vi "Parse ERD Write Expected Data.vi"(0 "Write ERD List":T1[](array[typedef]) {"ERD Number" format="%.0x"}, 11 "Error In":errorcluster) -> (8 "Expected Data":string, 15 "Error Out":errorcluster)   [LabVIEW 2023]
uses:
  type defs/ERD Write Data In.ctl
  type defs/Data Type.ctl
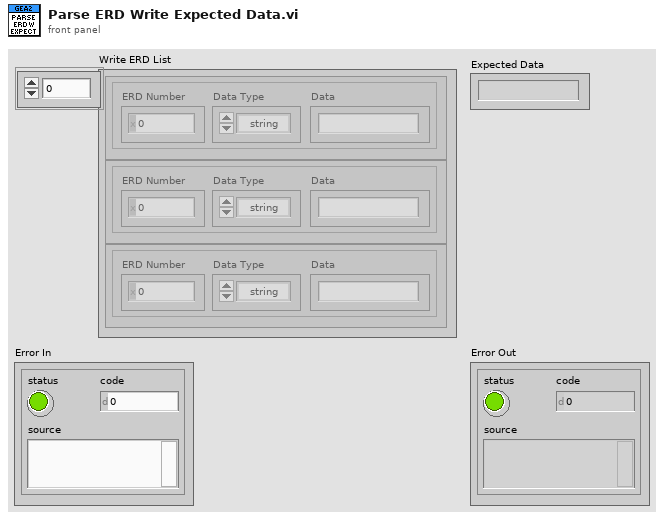
[diagram p1: front panel]
types:
  T1 = typedef "ERD Write Data In.ctl" = cluster{"ERD Number":u16, "Data Type":T2, "Data":string}
  T2 = typedef "Data Type.ctl" = enum16{"string", "boolean", "uint8_t", "uint16_t", "uint32_t", "uint64_t", "int8_t", "int16_t", "int32_t", "int64_t"}
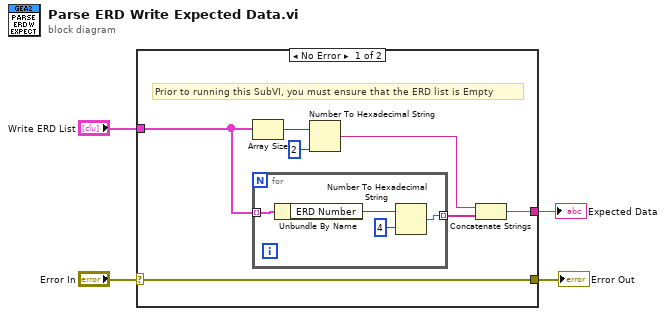
[diagram p0: block diagram]
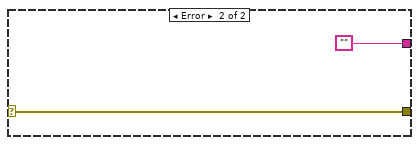
[diagram p2: hidden frame]
diagram:
  n1 = case shown="No Error" "Error In" {
    selector: "Error In" -> [w5 w17]
    tunnel: [w8 ""] -> w4
    tunnel: "Write ERD List" -> [w6 _]
    tunnel: [w5 w17] -> w2
    frame No Error {
      # "Prior to running this SubVI, you must ensure that the ERD list is Empty"
      n2 = Array Size(array=w6) -> (size(s)=w10:i32)
      n3 = for {
        tunnel: w6 -> [w15] mode=indexing
        tunnel: [w12] -> w11 mode=indexing
        n4 = Unbundle By Name(w15) -> ("ERD Number"=w14:u16)
        n5 = Number To Hexadecimal String(1:i16 4 ("width (-)"), 2:w14) -> (0:w12:string)
      }
      n6 = Number To Hexadecimal String(1:i16 2 ("width (-)"), 2:w10) -> (0:w7:string)
      n7 = Concatenate Strings(w7, w11) -> (w8:string)
    }
    frame Error {
    }
  }
  "Expected Data" <- w4
  "Error Out" <- w2
